vi "Auto Turn v2.vi"(9 "Orientation Angle":dbl=25.0) -> (3 "Done":bool)   [LabVIEW 2017]
uses:
  Robot Global Data.vi
  <vilib>/addons/control/pid/pid.llb/PID (DBL).vi
  <vilib>/addons/control/pid/NI_PID_pid.lvlib
panel:
  out "Turn Output":dbl=-0.003149999059550518 format="%.2f"
  out "Last 10 Compare Values":bool[](array[boolean])=[TRUE, FALSE, FALSE, FALSE, TRUE, TRUE, FALSE, FALSE, FALSE, FALSE]
  out "Gyro":dbl(graph)=23.89
  in  "PID gains - Angle":T1={"proportional gain (Kc)"=0.015, "integral time (Ti, min)"=0.0, "derivative time (Td, min)"=0.0022} {"derivative time (Td, min)" step=0.001 format="%.5f"; "integral time (Ti, min)" step=0.001 format="%.5f"; "proportional gain (Kc)" step=0.001 format="%.5f"}
  in  "Allowed Error":dbl=0.1
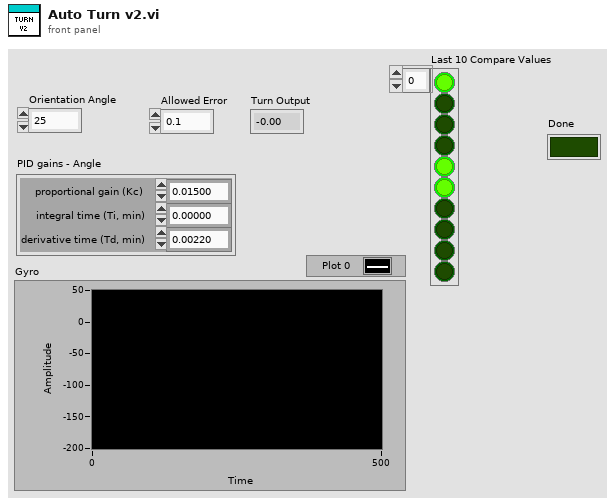
[diagram p1: front panel]
types:
  T1 = cluster{"proportional gain (Kc)":dbl, "integral time (Ti, min)":dbl, "derivative time (Td, min)":dbl}
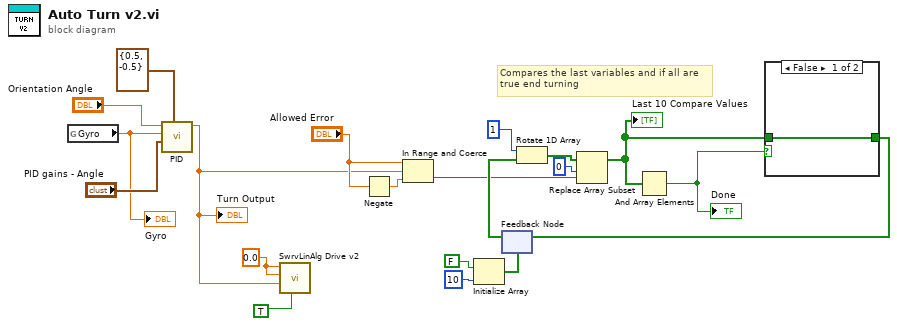
[diagram p0: block diagram]
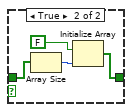
[diagram p2: hidden frame]
diagram:
  w7 = 0.0 ("X")
  # "Compares the last variables and if all are\ntrue end turning"
  n1 = global read "Robot Global Data.vi" "Gyro"() -> (w6:dbl)
  "Gyro" <- w6
  n2 = call-poly <vilib>:"PID.vi"("output range"=cluster{"output high":dbl, "output low":dbl} {"output high"=0.5, "output low"=-0.5}, "PID gains"="PID gains - Angle", "process variable"=w6, "setpoint"="Orientation Angle") -> ("output"=w1:dbl)  [unwired: 6 in, 1 out]
  "Turn Output" <- w1
  n3 = call "SwrvLinAlg Drive v2.vi"("Auto Controls"=TRUE, "Z"=w1, "Y"=w7, "X"=w7) -> ()  [unwired: 8 in]
  n4 = Negate(x="Allowed Error") -> (-x=w4:dbl)
  n5 = In Range and Coerce(upper limit="Allowed Error", x=w1, lower limit=w4) -> (In Range?=w12:bool)  [unwired: 1 out]
  n6 = Initialize Array(FALSE, 10 ("dimension size")) -> (w10:bool[])
  n7 = feedback #1(w10) -> (w14:bool[])
  n8 = Rotate 1D Array(1:w14, 2:1 ("n")) -> (0:w16:bool[])
  n9 = Replace Array Subset(array=w16, new element=w12, index=0) -> (w11:bool[])
  "Last 10 Compare Values" <- w11
  n10 = And Array Elements(Boolean array=w11) -> (logical AND=w2:bool)
  "Done" <- w2
  n11 = case shown="False" w2 {
    tunnel: w11 -> [w21 w23]
    tunnel: [w21 w22] -> w13
    frame False {
    }
    frame True {
      n12 = Array Size(array=w23) -> (size(s)=w24:i32)
      n13 = Initialize Array(FALSE, w24) -> (w22:bool[])
    }
  }
  n14 = feedback-in #1(w13) -> ()
